vi "Test Signal Channel.vi"(8 "error in (no error)":errorcluster, 11 "SR7270 Drivers in":refnum<class "SR7270 Drivers.lvclass">) -> (0 "error out":errorcluster, 3 "SR7270 Drivers out":refnum<class "SR7270 Drivers.lvclass">)   [LabVIEW 2016, in "SR7270 Drivers.lvlib"]
uses:
  SR7270 Drivers.lvlib
  <vilib>/addons/_JKI Toolkits/Caraya/classes/Test/Test.lvclass
  SR7270 Drivers.lvclass
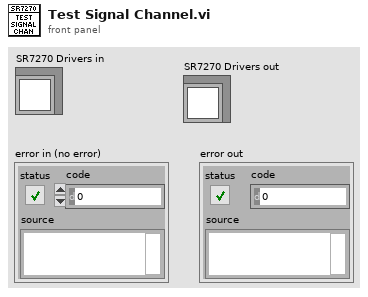
[diagram p1: front panel]
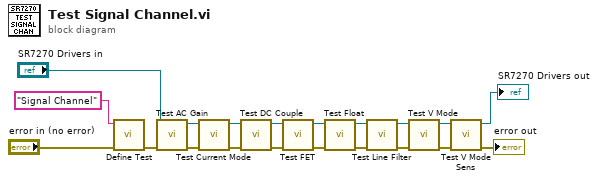
[diagram p0: block diagram]
diagram:
  n1 = call <vilib>:"Define Test.vi"("error in (no error)"="error in (no error)", "Label (VI Title)"="Signal Channel") -> ("error out"=w20:errorcluster)  [unwired: 9 in]
  n2 = call "Test AC Gain.vi"("error in (no error)"=w20, "SR7270 Drivers in"="SR7270 Drivers in") -> ("error out"=w3:errorcluster, "SR7270 Drivers out"=w2:refnum<class "SR7270 Drivers.lvclass">)  [unwired: 8 in]
  n3 = call "Test Current Mode.vi"("error in (no error)"=w3, "SR7270 Drivers in"=w2) -> ("error out"=w5:errorcluster, "SR7270 Drivers out"=w4:refnum<class "SR7270 Drivers.lvclass">)  [unwired: 8 in]
  n4 = call "Test DC Couple.vi"("error in (no error)"=w5, "SR7270 Drivers in"=w4) -> ("error out"=w7:errorcluster, "SR7270 Drivers out"=w6:refnum<class "SR7270 Drivers.lvclass">)  [unwired: 8 in]
  n5 = call "Test FET.vi"("error in (no error)"=w7, "SR7270 Drivers in"=w6) -> ("error out"=w9:errorcluster, "SR7270 Drivers out"=w8:refnum<class "SR7270 Drivers.lvclass">)  [unwired: 8 in]
  n6 = call "Test Float.vi"("error in (no error)"=w9, "SR7270 Drivers in"=w8) -> ("error out"=w10:errorcluster, "SR7270 Drivers out"=w13:refnum<class "SR7270 Drivers.lvclass">)  [unwired: 8 in]
  n7 = call "Test Line Filter.vi"("error in (no error)"=w10, "SR7270 Drivers in"=w13) -> ("error out"=w11:errorcluster, "SR7270 Drivers out"=w14:refnum<class "SR7270 Drivers.lvclass">)  [unwired: 8 in]
  n8 = call "Test V Mode.vi"("error in (no error)"=w11, "SR7270 Drivers in"=w14) -> ("error out"=w12:errorcluster, "SR7270 Drivers out"=w15:refnum<class "SR7270 Drivers.lvclass">)  [unwired: 8 in]
  n9 = call "Test V Mode Sens.vi"("error in (no error)"=w12, "SR7270 Drivers in"=w15) -> ("error out"=→"error out":errorcluster, "SR7270 Drivers out"=→"SR7270 Drivers out":refnum<class "SR7270 Drivers.lvclass">)  [unwired: 8 in]
